vi "Write ViewableActor Enqueuers.vi"(8 "error in (no error)":errorcluster, 10 "ViewableActor Enqueuers":refnum<class "Message Enqueuer.lvclass">[](array[class]), 11 "SubPanel Grid View in":refnum<class "SubPanel Grid View.lvclass">) -> (0 "error out":errorcluster, 3 "SubPanel Grid View out":refnum<class "SubPanel Grid View.lvclass">)   [LabVIEW 2012, in "Win8uiDemo.lvlib" / "SubPanel Grid View.lvclass"]
uses:
  SubPanel Grid View.lvclass
  <vilib>/ActorFramework/Message Enqueuer/Message Enqueuer.lvclass
  SubPanel Grid View.lvclass/SubPanel Grid View.ctl
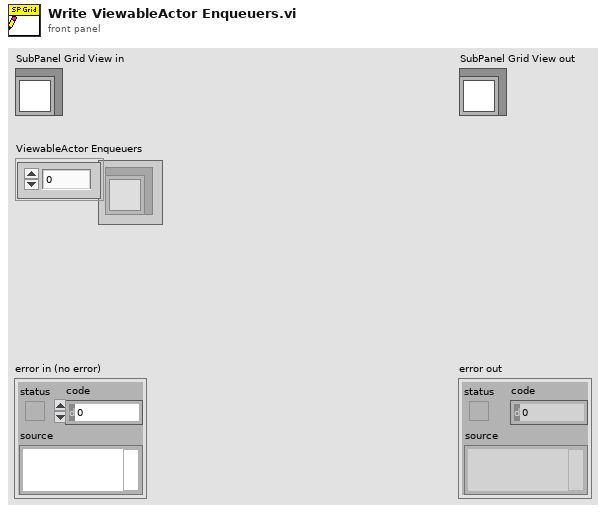
[diagram p1: front panel]
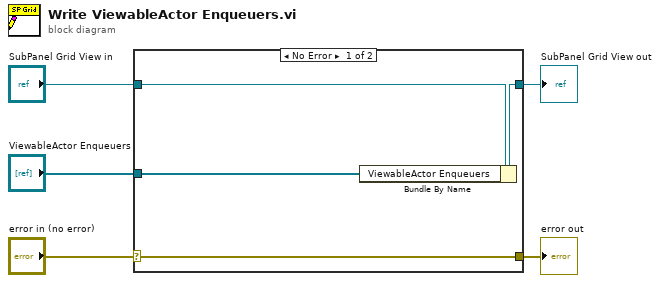
[diagram p0: block diagram]
diagram:
  n1 = case shown="No Error" "error in (no error)" {
    selector: "error in (no error)" -> [w9 w10]
    tunnel: [w9 w10] -> w4
    tunnel: [w7 w11] -> w2
    tunnel: "SubPanel Grid View in" -> [w8 w11]
    tunnel: "ViewableActor Enqueuers" -> [w6 _]
    frame No Error {
      n2 = Bundle By Name(cluster=w8, "ViewableActor Enqueuers"=w6) -> (w7:refnum<class "SubPanel Grid View.lvclass">)
    }
    frame Error {
    }
  }
  "error out" <- w4
  "SubPanel Grid View out" <- w2
